vi "GetReference2.vi"(0 "DeviceType":u32, 5 "DeviceInd":u32, 7 "CANInd":u32, 9 "RefType":T1 items=["REFTYPE_MODE"=0, "REFTYPE_FILTER"=1, "REFTYPE_ACR0"=2, "REFTYPE_AMR0"=6, "REFTYPE_kCANBAUD"=10, "REFTYPE_CANRX_EN"=13, "REFTYPE_UARTBAUD"=14, "REFTYPE_ALL"=15, "REFTYPE_BRS"=16], 11 "error in (no error)":errorcluster caption="错误输入（无错误）") -> (4 "Success":bool, 6 "Param":T2 {"ACR0" format="%x"}, 15 "error out":errorcluster caption="错误输出")   [LabVIEW 2011]
uses:
  VIs/Param.ctl
  VIs/ParamType.ctl
  data/ControlCAN.dll
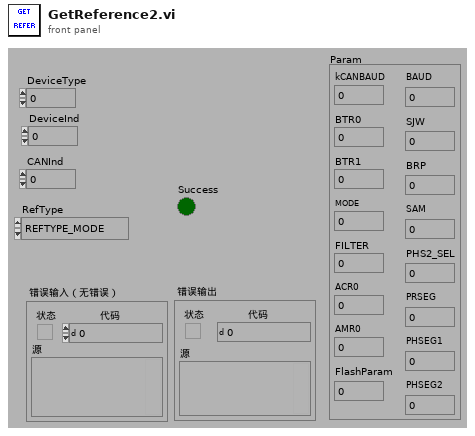
[diagram p1: front panel]
types:
  T1 = typedef "ParamType.ctl" = u32
  T2 = typedef "Param.ctl" = cluster{"kCANBAUD":u8, "BTR0":u8, "BTR1":u8, "MODE":u8, "FILTER":u8, "ACR0":u32, "AMR0":u32, "FlashParam":u32, "BAUD":u32, "SJW":u8, "BRP":u8, "SAM":u8, "PHS2_SEL":u8, "PRSEG":u8, "PHSEG1":u8, "PHSEG2":u8}
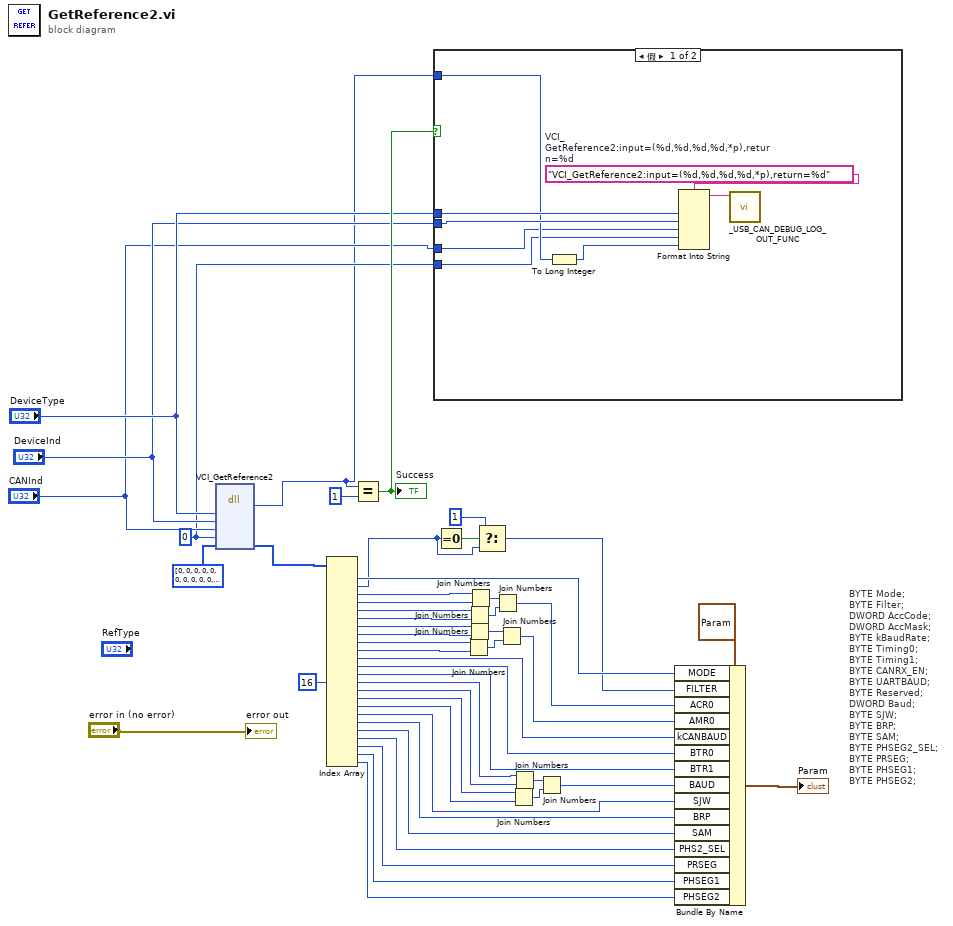
[diagram p0: block diagram]
diagram:
  w2 = u32 0 ("RefType")
  # "BYTE Mode;\t\t\t\nBYTE Filter;\t\t\nDWORD AccCode;\t\nDWORD AccMask;\t\nBYTE kBaudRate;\t\nBYTE Timing0;   \nBYTE Timing1;   \nBYTE CANRX_EN;\t\nBYTE UARTBAUD;\t\nBYTE Reserved;\nDWORD Baud;\t\t\t\nBYTE SJW;\t\t\t\t\nBYTE BRP;\t\t\t\t\nBYTE SAM;\t\t\t\t\nBYTE PHSEG2_SEL;\nBYTE PRSEG;\t\t\t\nBYTE PHSEG1;\t\t\nBYTE PHSEG2;"
  n1 = dll-call lib="PTH1Mabs ZHost_E工作TnewcodeUSB CAN Tool1.97dataControlCAN.dll" fn="VCI_GetReference2" label="VCI_GetReference"("DeviceType"="DeviceType", "DeviceInd"="DeviceInd", "CANInd"="CANInd", "RefType"=w2, "pData"=u8[] [0, 0, 0, 0, 0, 0, 0, 0, 0, 0, 0, 0, 0, 0, 0, 0, 0, 0, 0, 0, 0, 0, 0, 0, 0, 0, 0, 0, 0, 0, 0, 0]) -> ("返回类型"=w1:u32, "pData"=w46:u8[])  [unwired: 7 in, 2 out]
  n2 = Index Array(array=w46, index #14=16 ("索引")) -> (element #1=w41:u8, element #2=w9:u8, element #3=w38:u8, element #4=w37:u8, element #5=w36:u8, element #6=w35:u8, element #7=w31:u8, element #8=w30:u8, element #9=w29:u8, element #10=w28:u8, element #11=w26:u8, element #12=w25:u8, element #13=w24:u8, element #14=w22:u8, element #15=w21:u8, element #16=w20:u8, element #17=w19:u8, element #18=w17:u8, element #19=w16:u8, element #20=w15:u8, element #21=w14:u8, element #22=w13:u8, element #23=w12:u8, element #24=w11:u8)  [unwired: 23 in]
  n3 = Equal?(x=w1, y=u32 1) -> (x = y?=w6:bool)
  "Success" <- w6
  n4 = case shown="假" w6 {
    tunnel: "DeviceType" -> [w56 _]
    tunnel: "DeviceInd" -> [w55 _]
    tunnel: w1 -> [w54 _]
    tunnel: "CANInd" -> [w53 _]
    tunnel: w2 -> [w52 _]
    frame False {
      w50 = "VCI_GetReference2:input=(%d,%d,%d,%d,*p),return=%d"  # VCI_GetReference2:input=(%d,%d,%d,%d,*p),return=%d
      n5 = To Long Integer(number=w54) -> (32bit integer=w51:i32)
      n6 = Format Into String(format string=w50, w56, w55, w53, w52, w51) -> (resulting string=w57:string)  [unwired: 2 in, 1 out]
      n7 = call "_USB_CAN_DEBUG_LOG_OUT_FUNC.vi"("Info"=w57) -> ()  [unwired: 11 in]
    }
    frame True {
    }
  }
  n8 = Equal To 0?(x=w9) -> (x = 0?=w10:bool)
  n9 = Join Numbers(hi=w29, lo=w28) -> ((hi.lo)=w32:u16)
  n10 = Join Numbers(hi=w36, lo=w35) -> ((hi.lo)=w40:u16)
  n11 = Join Numbers(hi=w31, lo=w30) -> ((hi.lo)=w33:u16)
  n12 = Join Numbers(hi=w38, lo=w37) -> ((hi.lo)=w39:u16)
  n13 = Select(t=u8 1, s=w10, f=w9) -> (s? t:f=w7:u8)
  n14 = Join Numbers(hi=w39, lo=w40) -> ((hi.lo)=w34:u32)
  n15 = Join Numbers(hi=w33, lo=w32) -> ((hi.lo)=w27:u32)
  n16 = Join Numbers(hi=w20, lo=w19) -> ((hi.lo)=w42:u16)
  n17 = Join Numbers(hi=w22, lo=w21) -> ((hi.lo)=w43:u16)
  n18 = Join Numbers(hi=w43, lo=w42) -> ((hi.lo)=w18:u32)
  n19 = Bundle By Name(cluster=T2 {"kCANBAUD"=0, "BTR0"=0, "BTR1"=0, "MODE"=0, "FILTER"=0, "ACR0"=0, "AMR0"=0, "FlashParam"=0, "BAUD"=0, "SJW"=0, "BRP"=0, "SAM"=0, "PHS2_SEL"=0, "PRSEG"=0, "PHSEG1"=0, "PHSEG2"=0} ("Param 2"), "MODE"=w41, "FILTER"=w7, "ACR0"=w34, "AMR0"=w27, "kCANBAUD"=w26, "BTR0"=w25, "BTR1"=w24, "BAUD"=w18, "SJW"=w17, "BRP"=w16, "SAM"=w15, "PHS2_SEL"=w14, "PRSEG"=w13, "PHSEG1"=w12, "PHSEG2"=w11) -> (→"Param":T2)
  "error out" <- "error in (no error)"
